vi "ATF - DD Datalog and display modified.vi"() -> ()   [LabVIEW 2022 SP3]
doc: "Datalog and display software modified"
uses:
  Source Code/Control/SeCrTs-Enum.ctl
  Source Code/Globals/SeCrTS-DD globals.vi
panel:
  out "Backlog Storage":u64
  out "Backlog Pump":u64
  out "Logging Mode":string
  out "cmd":bool=TRUE
  out "Storage Connected?":bool
  in  "Pump IP Address":string="169.254.219.4"
  in  "Storage IP Address":string="169.254.219.4"
  out "Datalog Title":string
  in  "Exit":bool
  out "Log Period(Min)":dbl
  out "Logging?":bool
  out "Pumb Connected?":bool
  out "error Out":errorcluster
  # "ATF PUMP AND STORAGE"
  # "DATALOG REDUNDANT"
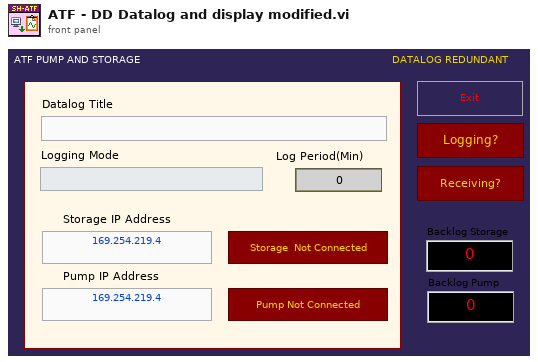
[diagram p1: front panel]
types:
  T1 = typedef "SeCrTs-Enum.ctl" = enum16{"Initialize", "Poll", "Establish ref", "Read", "Close", "Exit"}
  T2 = typedef "SeCrTS-Notifier Ref.ctl" = cluster{"DO NOT S":refnum<notifier>, "AI V NOT P":refnum<notifier>, "AI C NOT S":refnum<notifier>, "TC NOT P":refnum<notifier>, "DI NOT S":refnum<notifier>, "DI NOT P":refnum<notifier>, "DO NOT P":refnum<notifier>, "AI C NOT  P":refnum<notifier>}
  T3 = enum8{"Enabled", "Disabled", "Disabled and Grayed Out"}
  T4 = cluster{"C/NC":bool, "Start/Stop Log":bool[], "Log Name":string, "Config":cluster{"AO config":cluster{"Channel_Name":string, "Channel_Number":string, "Default_Value":dbl, "Units":string}[], "AI config":cluster{"Channel_Name":string, "Channel_Number":string, "Pre_Scale_min":dbl, "Pre_Scale_max":dbl, "Sensor_min":dbl, "Sensor_max":dbl, "Units":string}[], "DI config":cluster{"Channel_Name":string, "Channel_Number":string, "Default_Value":bool, "DI invert?":bool}[], "DO config":cluster{"Channel_Name":string, "Channel_Number":string, "Default_Value":bool, "DO invert?":bool}[], "TC config":cluster{"Channel_Name":string, "Channel_Number":string, "Pre_Scale_min":dbl, "Pre_Scale_max":dbl, "units":i32, " type":i32}[], "ACC config":cluster{"Channel_Name":string, "Channel_Number":string, "Pre_Scale_min":dbl, "Pre_Scale_max":dbl, "Terminal configuration":i32, "Sensitivity":dbl, "Sensitivity units":i32}[], "SG config":cluster{"Channel_Name":string, "Channel_Number":string, "Pre_Scale_min":dbl, "Pre_Scale_max":dbl}[], "Strain Gauge Settings":cluster{"poisson ratio":dbl, "nominal gage resistance":dbl, "gage factor":dbl}, "Bridge Settings":cluster{"voltage excitation value":dbl, "voltage excitation source":i32, "initial bridge voltage":dbl, "lead wire resistance":dbl, "strain configuration":i32}, "Sample Rate":cluster{"AI Sample Rate":dbl[], "AO Sample Rate":dbl[], "DI Sample Rate":dbl[], "TC Sample Rate":dbl[], "DO Sample Rate":dbl[], "SG Sample Rate":dbl[], "ACC Sample Rate":dbl[]}}, "Log min":dbl}
  T5 = cluster{"AO config":cluster{"Channel_Name":string, "Channel_Number":string, "Default_Value":dbl, "Units":string}[], "AI config":cluster{"Channel_Name":string, "Channel_Number":string, "Pre_Scale_min":dbl, "Pre_Scale_max":dbl, "Sensor_min":dbl, "Sensor_max":dbl, "Units":string}[], "DI config":cluster{"Channel_Name":string, "Channel_Number":string, "Default_Value":bool, "DI invert?":bool}[], "DO config":cluster{"Channel_Name":string, "Channel_Number":string, "Default_Value":bool, "DO invert?":bool}[], "TC config":cluster{"Channel_Name":string, "Channel_Number":string, "Pre_Scale_min":dbl, "Pre_Scale_max":dbl, "units":i32, " type":i32}[], "ACC config":cluster{"Channel_Name":string, "Channel_Number":string, "Pre_Scale_min":dbl, "Pre_Scale_max":dbl, "Terminal configuration":i32, "Sensitivity":dbl, "Sensitivity units":i32}[], "SG config":cluster{"Channel_Name":string, "Channel_Number":string, "Pre_Scale_min":dbl, "Pre_Scale_max":dbl}[], "Strain Gauge Settings":cluster{"poisson ratio":dbl, "nominal gage resistance":dbl, "gage factor":dbl}, "Bridge Settings":cluster{"voltage excitation value":dbl, "voltage excitation source":i32, "initial bridge voltage":dbl, "lead wire resistance":dbl, "strain configuration":i32}, "Sample Rate":cluster{"AI Sample Rate":dbl[], "AO Sample Rate":dbl[], "DI Sample Rate":dbl[], "TC Sample Rate":dbl[], "DO Sample Rate":dbl[], "SG Sample Rate":dbl[], "ACC Sample Rate":dbl[]}}
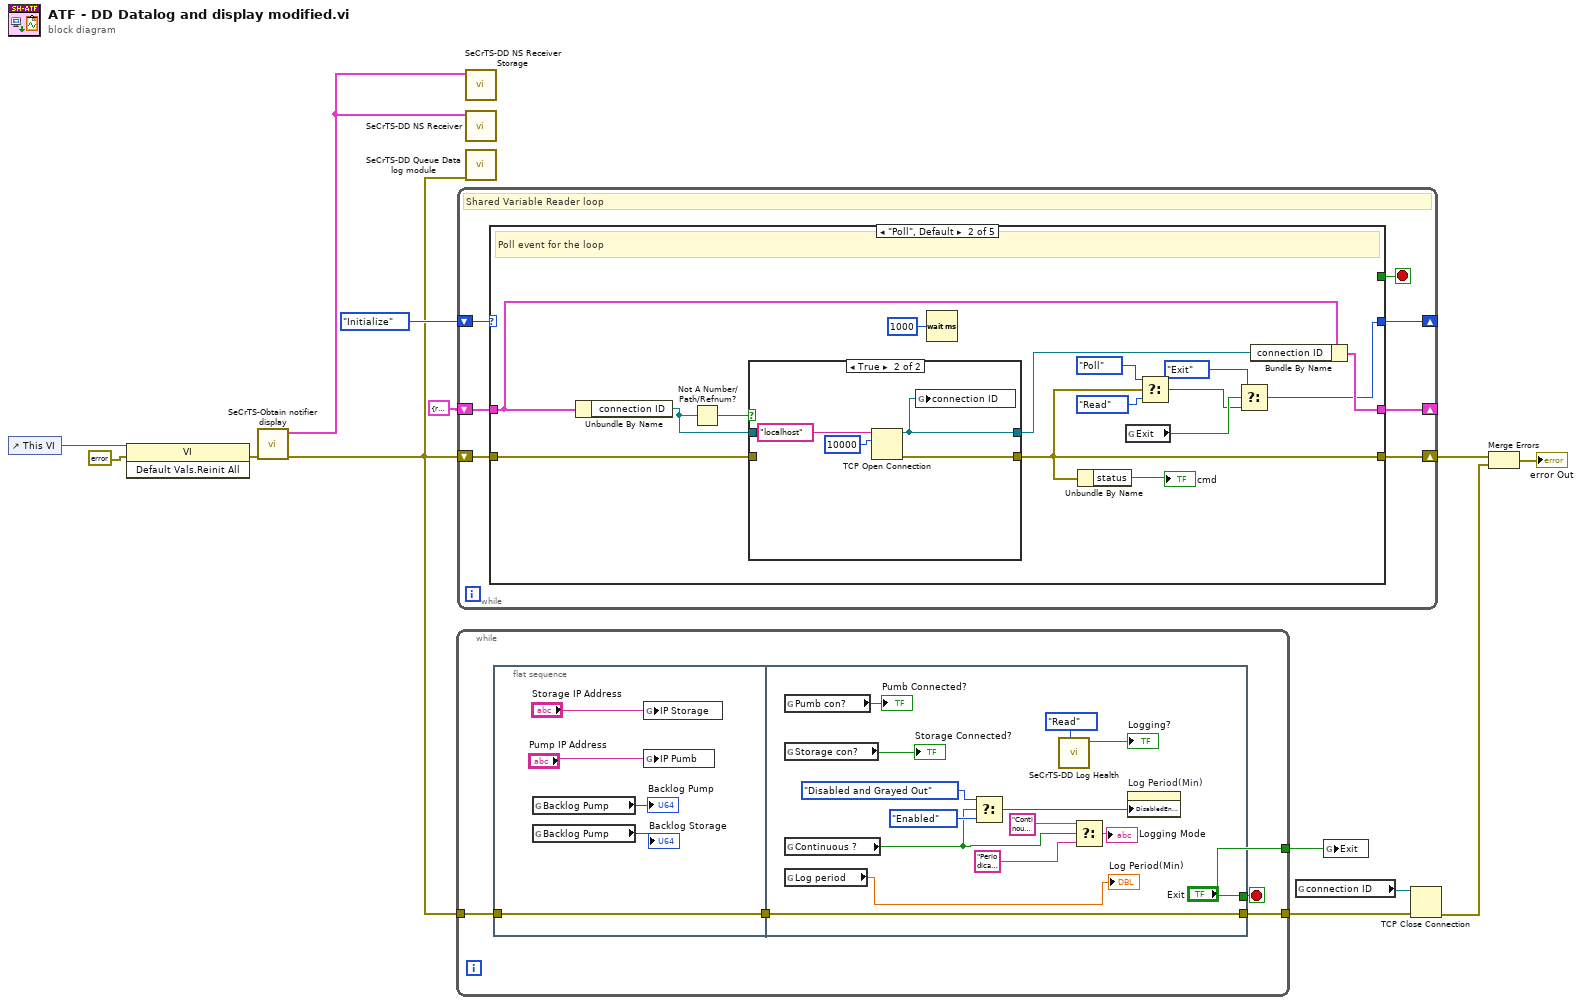
[diagram p0: block diagram]
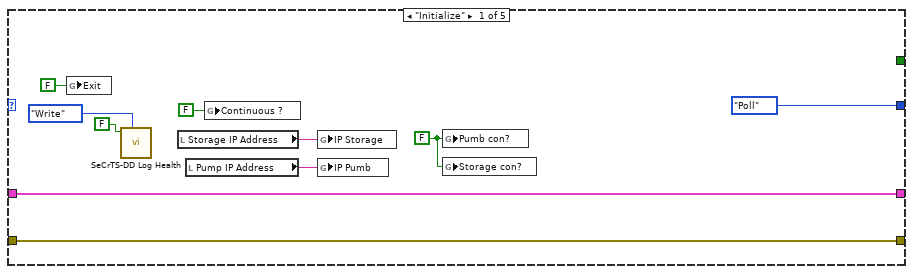
[diagram p2: hidden frame]
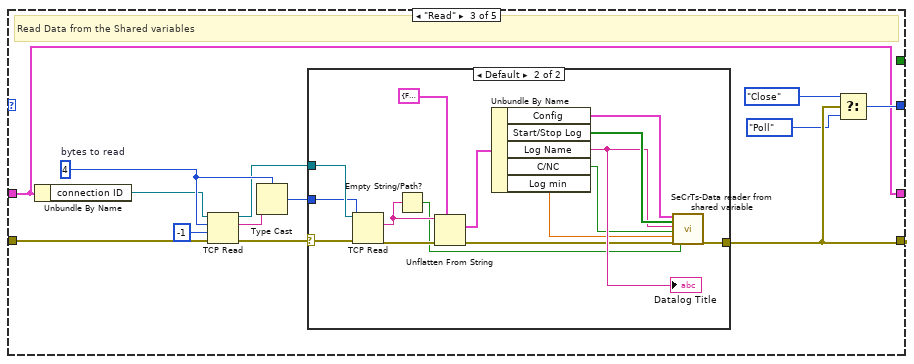
[diagram p4: hidden frame]
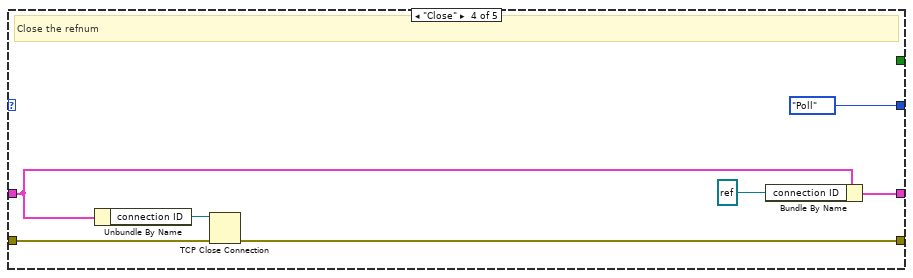
[diagram p6: hidden frame]
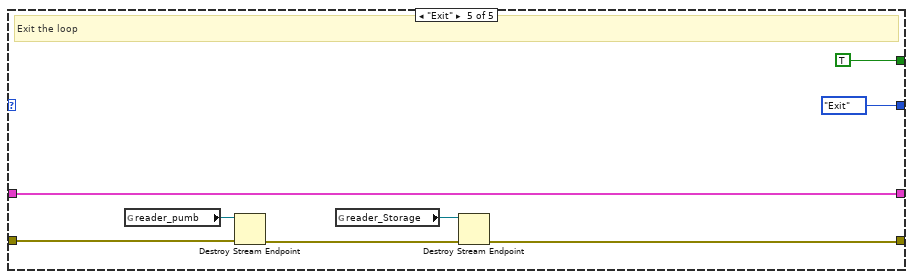
[diagram p7: hidden frame]
diagram:
  n1 = control-ref of="This VI"() -> (w12:refnum<vi>)
  n2 = invoke class="VI" method="Default Vals.Reinit All"(reference=w12, error in=errorcluster {"status"=FALSE, "code"=0, "source"=""}) -> (error out=w5:errorcluster)  [unwired: 1 in, 2 out]
  n3 = call "SeCrTS-Obtain notifier display.vi"("error in (no error)"=w5) -> ("error out"=w4:errorcluster, "NOT DIS Out"=w3:T2)  [unwired: 9 in]
  n4 = while {
    tunnel: w4 -> [w17]
    tunnel: [w15] -> w9
    tunnel: [w14] -> w2
    stop <- w14 stop-if-true
    n5 = flat-sequence {
      tunnel: w17 -> [w21]
      tunnel: [w21] -> w16
      tunnel: w16 -> [w29]
      tunnel: [w29] -> w15
      tunnel: ["Exit"] -> w14
      frame #0 {
        n6 = global read "SeCrTS-DD globals.vi" "Backlog Pump"() -> (→"Backlog Pump":u64)
        n7 = global read "SeCrTS-DD globals.vi" "Backlog Pump"() -> (→"Backlog Storage":u64)
        n8 = global write "SeCrTS-DD globals.vi" "IP Storage"("Storage IP Address") -> ()
        n9 = global write "SeCrTS-DD globals.vi" "IP Pumb"("Pump IP Address") -> ()
      }
      frame #1 {
        n10 = global read "SeCrTS-DD globals.vi" "Pumb con?"() -> (→"Pumb Connected?":bool)
        n11 = global read "SeCrTS-DD globals.vi" "Storage con?"() -> (→"Storage Connected?":bool)
        n12 = global read "SeCrTS-DD globals.vi" "Continuous ?"() -> (w26:bool)
        n13 = global read "SeCrTS-DD globals.vi" "Log period"() -> (→"Log Period(Min)":dbl)
        n14 = Select(t=T3."Disabled and Grayed Out" ("Disabled"), s=w26, f=T3."Enabled" ("Disabled")) -> (s? t:f=w35:T3)
        n15 = call "SeCrTS-DD Log Health.vi"("Enum"=enum16{"Read", "Write"}."Read") -> ("Log health R"=→"Logging?":bool)  [unwired: 9 in, 1 out]
        n16 = Select(t="Continous Logging Enabled" ("Logging Mode"), s=w26, f="Periodical Logging Enabled" ("Logging Mode")) -> (s? t:f=→"Logging Mode":string)
        n17 = property on="Log Period(Min)" class="DigNum (strict)"("DisabledEnum"=w35) -> ()  [unwired: 2 in, 2 out]
      }
    }
  }
  n18 = while {
    shift-right: [w40] -> _
    shift-left: SeCrTs-Enum."Initialize" -> [w43]
    shift-right: [w38] -> _
    shift-left: cluster{"connection ID":refnum<k5>} {"connection ID"=refnum} -> [w39]
    shift-right: [w41] -> w8
    shift-left: w4 -> [w42]
    stop <- w37 stop-if-true
    # "Shared Variable Reader loop"
    n19 = case shown="\"Poll\", Default" w43 {
      tunnel: w42 -> [w44 w62 w84 w108 w113]
      tunnel: [w44 w63 w81 w107 w111] -> w41
      tunnel: [SeCrTs-Enum."Poll" w55 w78 SeCrTs-Enum."Poll" SeCrTs-Enum."Exit"] -> w40
      tunnel: w39 -> [w52 w67 w77 w105 w116]
      tunnel: [w52 w68 w77 w106 w116] -> w38
      tunnel: [_ _ _ _ TRUE] -> w37
      frame "Initialize" {
        w51 = FALSE ("Connect?")
        n20 = global write "SeCrTS-DD globals.vi" "Exit"(FALSE ("EXIT")) -> ()
        n21 = call "SeCrTS-DD Log Health.vi"("Enum"=enum16{"Read", "Write"}."Write", "Log health"=FALSE) -> ()  [unwired: 8 in, 2 out]
        n22 = local read "Storage IP Address"() -> (w50:string)
        n23 = local read "Pump IP Address"() -> (w46:string)
        n24 = global write "SeCrTS-DD globals.vi" "Continuous ?"(FALSE ("Continuous ?")) -> ()
        n25 = global write "SeCrTS-DD globals.vi" "IP Storage"(w50) -> ()
        n26 = global write "SeCrTS-DD globals.vi" "IP Pumb"(w46) -> ()
        n27 = global write "SeCrTS-DD globals.vi" "Pumb con?"(w51) -> ()
        n28 = global write "SeCrTS-DD globals.vi" "Storage con?"(w51) -> ()
      }
      frame "Poll", Default {
        # "Poll event for the loop"
        n29 = Unbundle By Name(w67) -> ("connection ID"=w65:refnum<k5>)
        n30 = Not A Number/Path/Refnum?(number/path/refnum=w65) -> (NaN/Path/Refnum?=w66:bool)
        n31 = case shown="True" w66 {
          tunnel: [w70 w71] -> w59
          tunnel: w65 -> [w70 _]
          tunnel: [w69 w74] -> w63
          tunnel: w62 -> [w69 _]
          frame False {
          }
          frame True {
            n32 = TCP Open Connection(address="localhost", remote port or service name=u16 10000) -> (connection ID=w71:refnum<k5>, error out=w74:errorcluster)  [unwired: 3 in]
            n33 = global write "SeCrTS-DD globals.vi" "connection ID"(w71) -> ()
          }
        }
        n34 = Wait (ms)(milliseconds to wait=u32 1000) -> ()  [unwired: 1 out]
        n35 = Unbundle By Name(w63) -> ("status"=→"cmd":bool)
        n36 = global read "SeCrTS-DD globals.vi" "Exit"() -> (w58:bool)
        n37 = Select(t=SeCrTs-Enum."Poll", s=w63, f=SeCrTs-Enum."Read") -> (s? t:f=w57:T1)
        n38 = Select(t=SeCrTs-Enum."Exit", s=w58, f=w57) -> (s? t:f=w55:T1)
        n39 = Bundle By Name(cluster=w67, "connection ID"=w59) -> (w68:cluster{"connection ID":refnum<k5>})
      }
      frame "Read" {
        w86 = 4  # bytes to read
        # "Read Data from the Shared variables"
        n40 = Unbundle By Name(w77) -> ("connection ID"=w83:refnum<k5>)
        n41 = TCP Read(connection ID=w83, bytes to read=w86, error in (no error)=w84, 9:-1 ("timeout ms (25000)")) -> (connection ID out=w82:refnum<k5>, data out=w87:string, error out=w76:errorcluster)  [unwired: 1 in]
        n42 = Type Cast(type=w86, x=w87) -> (*(type *) &x=w85:i32)
        n43 = case shown="Default" w76 {
          selector: w76 -> [w88 w102]
          tunnel: w82 -> [_ w103]
          tunnel: [w88 w89] -> w81
          tunnel: w85 -> [_ w101]
          frame #0 {
            # "The server has not written any data"
          }
          frame #1 {
            n44 = TCP Read(connection ID=w103, bytes to read=w101, error in (no error)=w102) -> (data out=w93:string, error out=w92:errorcluster)  [unwired: 2 in, 1 out]
            n45 = Empty String/Path?(string/path=w93) -> (empty?=w91:bool)
            n46 = Unflatten From String(type=T4 {"C/NC"=FALSE, "Start/Stop Log"=[], "Log Name"="", "Config"={"AO config"=[], "AI config"=[], "DI config"=[], "DO config"=[], "TC config"=[], "ACC config"=[], "SG config"=[], "Strain Gauge Settings"={"poisson ratio"=0.0, "nominal gage resistance"=0.0, "gage factor"=0.0}, "Bridge Settings"={"voltage excitation value"=0.0, "voltage excitation source"=0, "initial bridge voltage"=0.0, "lead wire resistance"=0.0, "strain configuration"=0}, "Sample Rate"={"AI Sample Rate"=[], "AO Sample Rate"=[], "DI Sample Rate"=[], "TC Sample Rate"=[], "DO Sample Rate"=[], "SG Sample Rate"=[], "ACC Sample Rate"=[]}}, "Log min"=0.0} ("Cluster"), binary string=w93, error in (no error)=w92) -> (value=w99:T4, error out=w90:errorcluster)  [unwired: 2 in, 1 out]
            n47 = Unbundle By Name(w99) -> ("Config"=w98:T5, "Start/Stop Log"=w97:bool[], "Log Name"=w96:string, "C/NC"=w95:bool, "Log min"=w94:dbl)
            "Datalog Title" <- w96
            n48 = call "SeCrTs-Data reader from shared variable.vi"("Config"=w98, "Start/Stop Log"=w97, "Log Name"=w96, "C/NC"=w95, "Log min"=w94, "error IO"=w90, "empty?"=w91) -> ("error out"=w89:errorcluster)  [unwired: 12 in]
          }
        }
        n49 = Select(t=SeCrTs-Enum."Close", s=w81, f=SeCrTs-Enum."Poll") -> (s? t:f=w78:T1)
      }
      frame "Close" {
        # "Close the refnum"
        n50 = Unbundle By Name(w105) -> ("connection ID"=w109:refnum<k5>)
        n51 = TCP Close Connection(connection ID=w109, error in (no error)=w108) -> (error out=w107:errorcluster)  [unwired: 1 in, 1 out]
        n52 = Bundle By Name(cluster=w105, "connection ID"=refnum<k5> refnum) -> (w106:cluster{"connection ID":refnum<k5>})
      }
      frame "Exit" {
        # "Exit the loop"
        n53 = global read "SeCrTS-DD globals.vi" "reader_pumb"() -> (w115:refnum<k21>)
        n54 = Destroy Stream Endpoint(8:w113, 11:w115) -> (0:w112:errorcluster)
        n55 = global read "SeCrTS-DD globals.vi" "reader_Storage"() -> (w114:refnum<k21>)
        n56 = Destroy Stream Endpoint(8:w112, 11:w114) -> (0:w111:errorcluster)
      }
    }
  }
  n57 = call "SeCrTS-DD NS Receiver Storage.vi"("NOT DIS Out"=w3) -> ()  [unwired: 11 in]
  n58 = call "SeCrTS-DD NS Receiver.vi"("NOT DIS Out"=w3) -> ()  [unwired: 11 in]
  n59 = call "SeCrTS-DD Queue Data log module.vi"("error in"=w4) -> ()  [unwired: 10 in, 1 out]
  n60 = global read "SeCrTS-DD globals.vi" "connection ID"() -> (w1:refnum<k5>)
  n61 = global write "SeCrTS-DD globals.vi" "Exit"(w2) -> ()
  n62 = TCP Close Connection(connection ID=w1, error in (no error)=w9) -> (error out=w6:errorcluster)  [unwired: 1 in, 1 out]
  n63 = Merge Errors(w8, w6) -> (→"error Out":errorcluster)
